vi "SPI Write Read Bytes.vi"(4 "IntervalTimeUs":i32, 5 "ReadLen":i32, 6 "pReadData":u8[](array[numeric])=array[4097 elements], 7 "WriteLen":i32, 9 "pWriteData":u8[](array[numeric])=array[4097 elements], 10 "SPIIndex":i32, 11 "DevHandle":i32) -> (1 "pWriteData out":u8[](array[numeric]), 2 "function return":i32, 3 "pReadData out":u8[](array[numeric]))   [LabVIEW 2010, in "usb2spi.lvlib"]
doc: "int WINAPI SPI_WriteReadBytes(int DevHandle,int SPIIndex,unsigned char *pWriteData,int WriteLen,unsigned char *pReadData,int ReadLen,int IntervalTimeUs);"
uses:
  usb2spi.lvlib
  USB2XXX/trunk/USB2XXX/USB2XXX/vs2019/Release/USB2XXX.dll
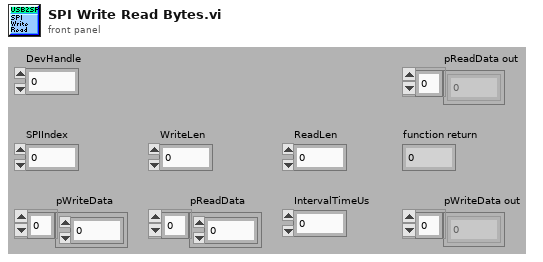
[diagram p1: front panel]
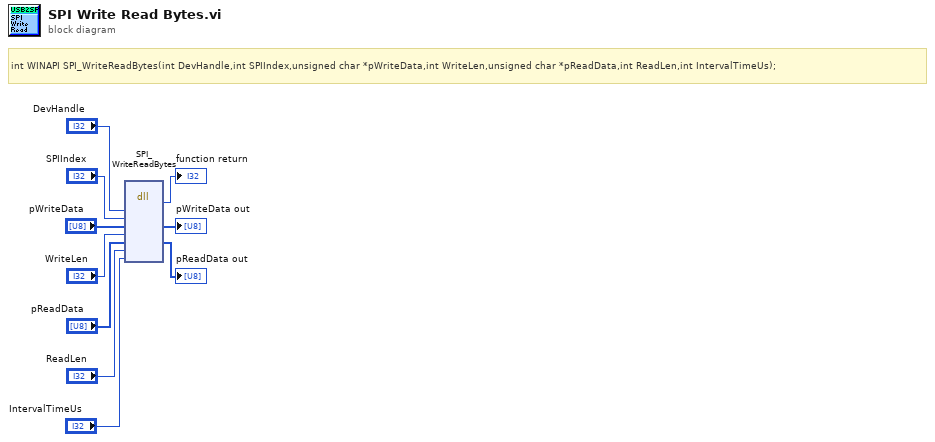
[diagram p0: block diagram]
diagram:
  # "int WINAPI SPI_WriteReadBytes(int DevHandle,int SPIIndex,unsigned char *pWriteData,int WriteLen,unsigned char *pReadData,int ReadLen,int IntervalTimeUs);"
  n1 = dll-call lib="E:/Projects/USB2XXX/trunk/USB2XXX/USB2XXX/vs2019/Release/USB2XXX.*" fn="SPI_WriteReadBytes"("DevHandle"="DevHandle", "SPIIndex"="SPIIndex", "pWriteData"="pWriteData", "WriteLen"="WriteLen", "pReadData"="pReadData", "ReadLen"="ReadLen", "IntervalTimeUs"="IntervalTimeUs") -> (→"function return":i32, "pWriteData"=→"pWriteData out":u8[], "pReadData"=→"pReadData out":u8[])  [unwired: 8 in, 2 out]
